vi "Analysatoren abgleichen.vi"(10 "Analysatorliste":string[](array[string]), 11 "Analysatoren":string[](array[string])) -> (3 "x != y?":bool)   [LabVIEW 2020, in "System Einstellungen V2.lvlib"]
uses:
  System Einstellungen V2.lvlib
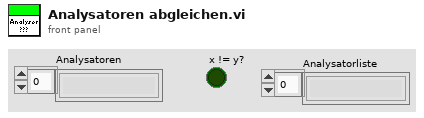
[diagram p1: front panel]
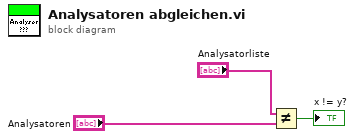
[diagram p0: block diagram]
diagram:
  n1 = Not Equal?(x="Analysatorliste", y="Analysatoren") -> (x != y?=→"x != y?":bool)
